vi "Etape4.vi"() -> ()   [LabVIEW 2020]
uses:
  <instrlib>/Agilent 34401/Public/Data/Read (Single Point).vi
  <instrlib>/Agilent E363X Series/Agilent E363X Series.lvlib
  <instrlib>/Agilent 34401/Agilent 34401.lvlib
panel:
  out "XY Graph":cluster{"Y":dbl[], "Y":dbl[]}[](graph) caption="Graphe XY"
  in  "Plage tension":dbl(slide) scale=0.0..6.0
  out "Courant":dbl
  in  "Incrément tension":dbl
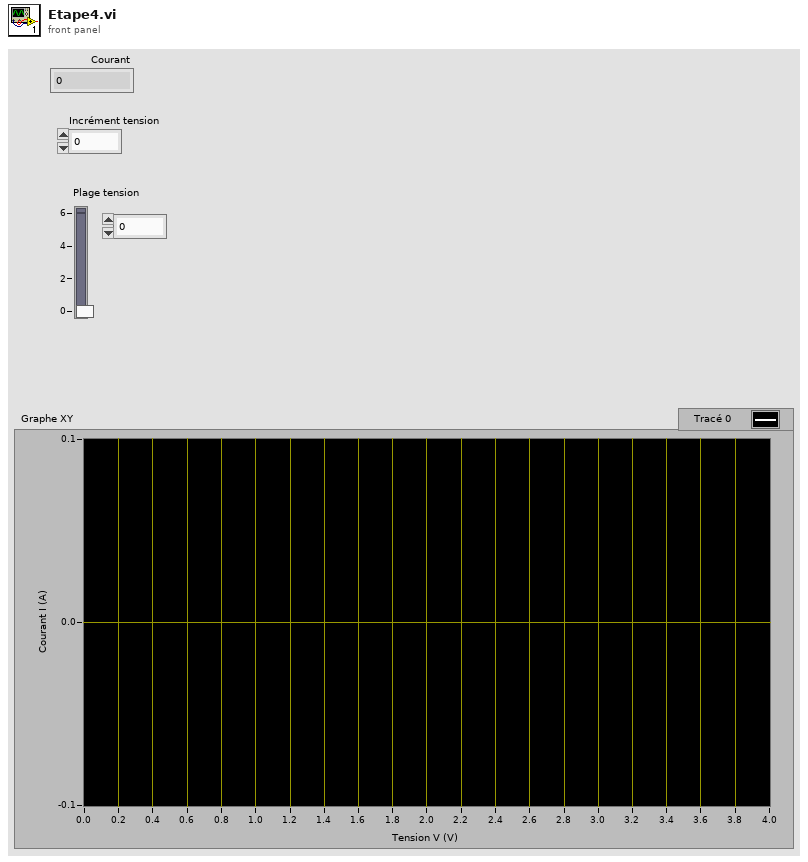
[diagram p1: front panel]
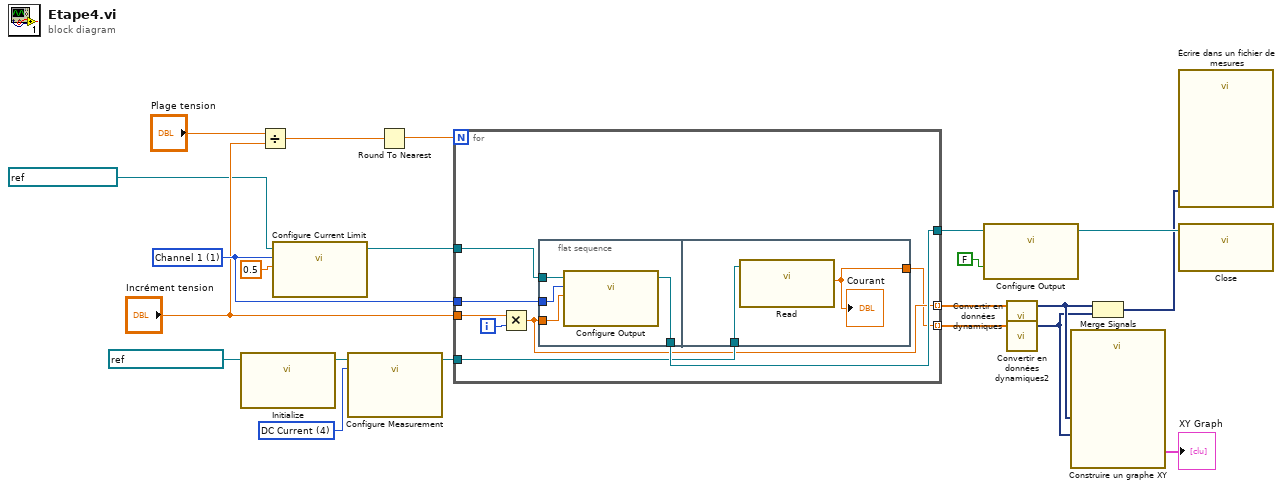
[diagram p0: block diagram]
diagram:
  w18 = u16 4 items=["DC Voltage", "AC Voltage", "2 - Wire Resistance", "4 - Wire Resistance", "DC Current", "AC Current", "Frequency", "Period", "Continuity", "Diode Checking", "VDC:VDC Ratio", "Temperature", "Capacitance"] ("Function (0: DC Voltage)")
  w14 = 1 items=["Channel 1"=1, "Channel 2"=2, "Channel 3"=3] ("Channel (1: Channel 1)")
  n1 = call <instrlib>:"Initialize.vi"("VISA resource name"=refnum<visa-resource-name> "GPIB0::22::INSTR") -> ("VISA resource name out"=w19:refnum<visa-resource-name>)  [unwired: 9 in, 1 out]
  n2 = Divide(x="Plage tension", y="Incrément tension") -> (x/y=w10:dbl)
  n3 = call <instrlib>:"Configure Current Limit.vi"("Current Limit (0.0 A)"=0.5, "Channel (1: Channel 1)"=w14, "VISA resource name"=refnum<visa-resource-name> "GPIB0::5::INSTR" ("VISA resource name out")) -> ("VISA resource name out"=w13:refnum<visa-resource-name>)  [unwired: 7 in, 1 out]
  n4 = call <instrlib>:"Configure Measurement.vi"("Function (0: DC Voltage)"=w18, "VISA resource name"=w19) -> ("VISA resource name out"=w15:refnum<visa-resource-name>)  [unwired: 8 in, 1 out]
  n5 = Round To Nearest(number=w10) -> (nearest integer value=w8:dbl)
  n6 = for {
    N: w8 -> [_]
    tunnel: w15 -> [w26]
    tunnel: w14 -> [w29]
    tunnel: w13 -> [w28]
    tunnel: [w27] -> w12
    tunnel: "Incrément tension" -> [w25]
    tunnel: [w23] -> w6 mode=indexing
    tunnel: [w22] -> w5 mode=indexing
    i -> [w24]
    n7 = Multiply(x=w25, y=w24) -> (x*y=w23:dbl)
    n8 = flat-sequence {
      tunnel: w29 -> [w33]
      tunnel: w28 -> [w32]
      tunnel: [w31] -> w27
      tunnel: w23 -> [w30]
      tunnel: w26 -> [w35]
      tunnel: [w34] -> w22
      frame #0 {
        n9 = call <instrlib>:"Configure Output.vi"("Voltage Level (0.0 V)"=w30, "Channel (1: Channel 1)"=w33, "VISA resource name"=w32) -> ("VISA resource name out"=w31:refnum<visa-resource-name>)  [unwired: 7 in, 1 out]
      }
      frame #1 {
        n10 = call-poly <instrlib>:"Read.vi"("VISA resource name"=w35) -> ("Measurement"=w34:dbl)  [unwired: 8 in, 2 out]
        "Courant" <- w34
      }
    }
  }
  n11 = call <instrlib>:"Configure Output.vi"("Enable Output (T: Enable)"=FALSE, "VISA resource name"=w12) -> ("VISA resource name out"=w16:refnum<visa-resource-name>)  [unwired: 8 in, 1 out]
  n12 = call "Convertir en données dynamiques"("Array"=w6) -> ("Dynamic Data Type"=w4:dynamicdata)  [unwired: 3 in]
  n13 = call "Convertir en données dynamiques2"("Array"=w5) -> ("Dynamic Data Type"=w3:dynamicdata)  [unwired: 3 in]
  n14 = call "Construire un graphe XY"("Y Input"=w3, "X Input"=w4) -> ("XY Graph"=→"XY Graph":cluster{"X":dbl[], "Y":dbl[]}[])  [unwired: 8 in, 1 out]
  n15 = Merge Signals(w4, w3) -> (w2:dynamicdata)
  n16 = call "Écrire dans un fichier de mesures"("Signals"=w2) -> ()  [unwired: 16 in, 3 out]
  n17 = call <instrlib>:"Close.vi"("VISA resource name"=w16) -> ()  [unwired: 10 in, 1 out]
